vi "Bookmarks View Shortcut Menu Activation.vi"(8 "Error In":errorcluster, 9 "Coords":T1, 10 "MenuRef":refnum<k9>, 11 "TreeControl In":refnum<vi>) -> (0 "Error Out":errorcluster, 3 "TreeControl Out":refnum<vi>)   [LabVIEW 2018, in "Bookmark Manager.lvlib"]
uses:
  Bookmark Manager.lvlib
  <vilib>/Utility/miscctls.llb/LVPoint32TypeDef.ctl
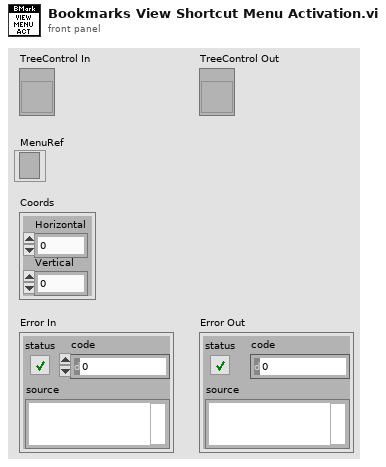
[diagram p1: front panel]
types:
  T1 = typedef "LVPoint32TypeDef.ctl" = cluster{"Horizontal":i32, "Vertical":i32}
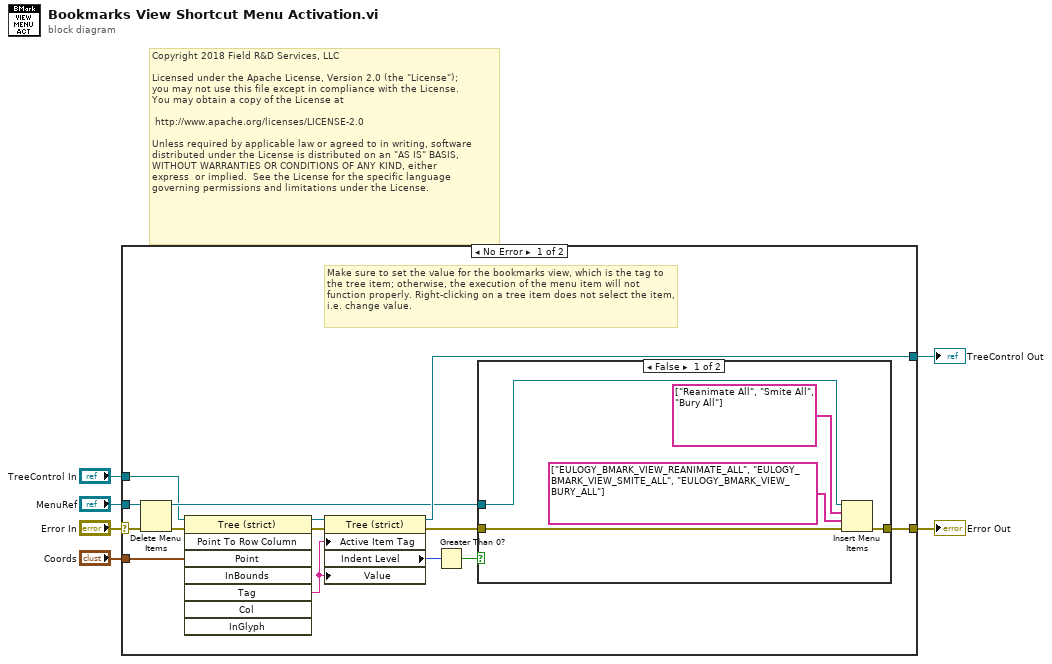
[diagram p0: block diagram]
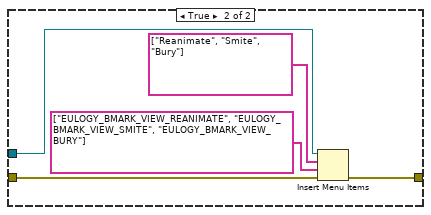
[diagram p2: hidden frame]
diagram:
  # "Copyright 2018 Field R&D Services, LLC\n\nLicensed under the Apache License, Version 2.0 (the \"License\");\nyou may not use this file except in compliance with the License.\nYou may obtain a copy of the License at\n\n\thttp://www.apache.org/licenses/LICENSE-2.0\n\nUnless required by applicable law or agreed to in writing, software\ndistributed under the License is distributed on an \"AS IS\" BASIS,\nWITHOUT WARRANTIES OR CONDITIONS OF ANY KIND, either \nexpress  or implied.  See the License for the specific language \ngoverning permissions and limitations under the License."
  n1 = case shown="No Error" "Error In" {
    selector: "Error In" -> [w7 w31]
    tunnel: [w19 w32] -> w6
    tunnel: [w18 w31] -> w5
    tunnel: "Coords" -> [w12 _]
    tunnel: "TreeControl In" -> [w9 w32]
    tunnel: "MenuRef" -> [w8 _]
    frame No Error {
      # "Make sure to set the value for the bookmarks view, which is the tag to the tree item; otherwise, the execution of the menu item will not function properly. Right-clicking on a tree item does not select the item, i.e. change value."
      n2 = Delete Menu Items(6:w7, 9:w8) -> (0:w11:errorcluster, 3:w17:refnum<k9>)  [unwired: 2 in]
      n3 = invoke class="Tree (strict)" method="Point To Row Column"(reference=w9, error in=w11, "Point"=w12) -> (reference out=w10:refnum<vi>, error out=w13:errorcluster, "Tag"=w20:string)  [unwired: 5 in, 5 out]
      n4 = property class="Tree (strict)"(reference=w10, error in=w13, "Active Item Tag"=w20, "Value"=w20) -> (reference out=w19:refnum<vi>, error out=w16:errorcluster, "Indent Level"=w14:i32)
      n5 = Greater Than 0?(x=w14) -> (x > 0?=w15:bool)
      n6 = case shown="False" w15 {
        tunnel: w16 -> [w23 w28]
        tunnel: w17 -> [w21 w27]
        tunnel: [w22 w26] -> w18
        frame False {
          n7 = Insert Menu Items(6:w23, 7:string[] ["EULOGY_BMARK_VIEW_REANIMATE_ALL", "EULOGY_BMARK_VIEW_SMITE_ALL", "EULOGY_BMARK_VIEW_BURY_ALL"] ("item tags"), 8:string[] ["Reanimate All", "Smite All", "Bury All"] ("item names"), 9:w21) -> (0:w22:errorcluster)  [unwired: 2 in, 2 out]
        }
        frame True {
          n8 = Insert Menu Items(6:w28, 7:string[] ["EULOGY_BMARK_VIEW_REANIMATE", "EULOGY_BMARK_VIEW_SMITE", "EULOGY_BMARK_VIEW_BURY"] ("item tags"), 8:string[] ["Reanimate", "Smite", "Bury"] ("item names"), 9:w27) -> (0:w26:errorcluster)  [unwired: 2 in, 2 out]
        }
      }
    }
    frame Error {
    }
  }
  "TreeControl Out" <- w6
  "Error Out" <- w5
